vi "Get Formula.vi"(4 "Make Formula":bool) -> (0 "Formula Made":bool, 1 "Cannon Angle Set Point":dbl, 2 "RPM Set Point":dbl)   [LabVIEW 2012]
uses:
  BotStatus.vi
  <vilib>/express/express arith-compare/Formula/XNode/ExpressFormulaBlockNode.xnode
panel:
  in  "Distance before starting":dbl
  in  "Angle before starting":dbl
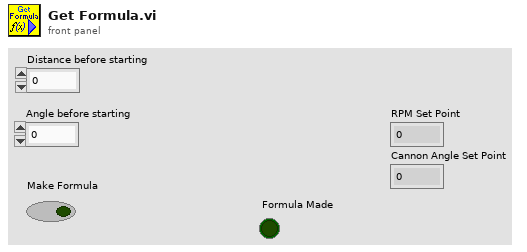
[diagram p1: front panel]
types:
  T1 = cluster{"Middle":bool, "InCannon":bool, "InFlipper":bool, "FlipperAtPlace":bool, "Bottom":bool, "FrisbeeDirection":bool}
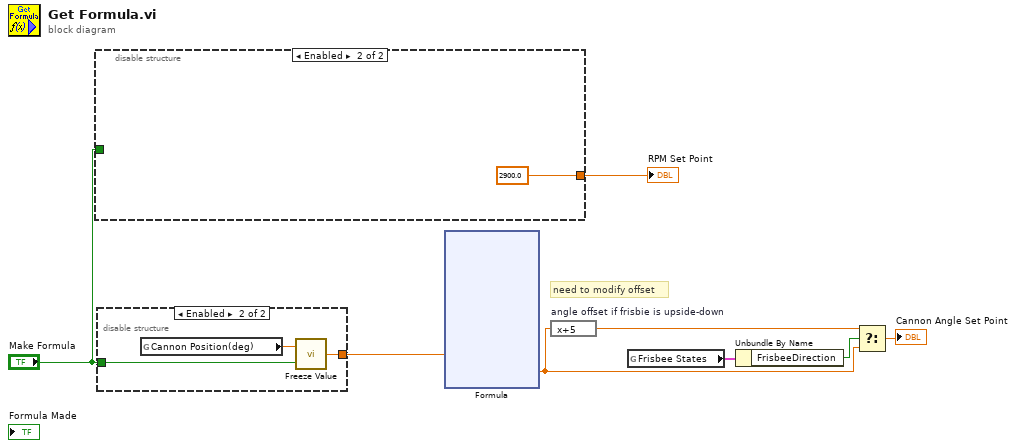
[diagram p0: block diagram]
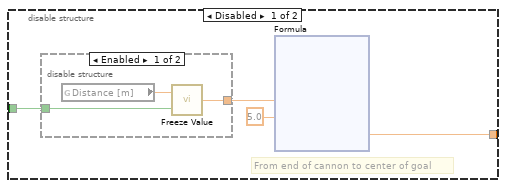
[diagram p2: hidden frame]
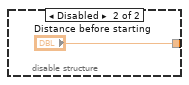
[diagram p3: hidden frame]
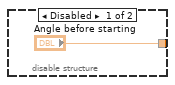
[diagram p4: hidden frame]
diagram:
  # "need to modify offset"
  n1 = disable-structure shown="Enabled" {
    disable-tunnel: [w12 2900.0 ("angle")] -> w4
    disable-tunnel: "Make Formula" -> [w10 _]
    frame Disabled {
      # "From end of cannon to center of goal"
      n2 = disable-structure shown="Enabled" {
        disable-tunnel: [w24 "Distance before starting"] -> w11
        disable-tunnel: w10 -> [w23 _]
        frame Enabled {
          n3 = global read "BotStatus.vi" "Distance [m]"() -> (w25:dbl)
          n4 = call "Freeze Value.vi"("Freeze Value"=w23, "In Value"=w25) -> ("Value Out"=w24:dbl)
        }
        frame Disabled {
        }
      }
      n5 = xnode "Formula"("D"=w11, "angle"=5.0) -> ("Result"=w12:dbl)  [unwired: 1 in, 1 out]
    }
    frame Enabled {
    }
  }
  "RPM Set Point" <- w4
  n6 = disable-structure shown="Enabled" {
    disable-tunnel: ["Angle before starting" w30] -> w2
    disable-tunnel: "Make Formula" -> [_ w29]
    frame Disabled {
    }
    frame Enabled {
      n7 = global read "BotStatus.vi" "Cannon Position(deg)"() -> (w31:dbl)
      n8 = call "Freeze Value.vi"("Freeze Value"=w29, "In Value"=w31) -> ("Value Out"=w30:dbl)
    }
  }
  n9 = xnode "Formula"("angle"=w2) -> ("Result"=w5:dbl)  [unwired: 4 in, 1 out]
  n10 = expression code="x+5" "angle offset if frisbie is upside-down"(w5) -> (w6:dbl)
  n11 = global read "BotStatus.vi" "Frisbee States"() -> (w7:T1)
  n12 = Unbundle By Name(w7) -> ("FrisbeeDirection"=w8:bool)
  n13 = Select(t=w6, s=w8, f=w5) -> (s? t:f=→"Cannon Angle Set Point":dbl)
